vi "Script Project FIFOs.vi"(7 "Number of SPI Buses":i32, 8 "error in (no error)":errorcluster, 9 "Device Channels":i32[](array[numeric]), 10 "LabVIEW Project to Script":path, 11 "Curent Bus Path":path) -> (0 "error out":errorcluster)   [LabVIEW 2014, in "Initialization and IO Node Scripting.lvlib"]
uses:
  Initialization and IO Node Scripting.lvlib
  State Machine/Controls/Values for Naming.ctl
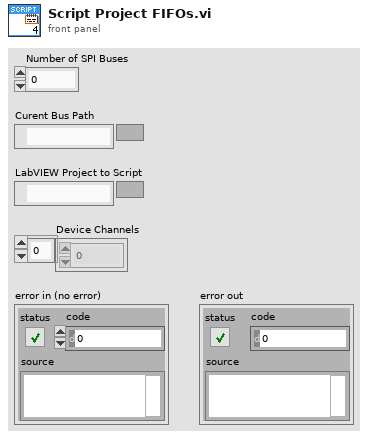
[diagram p1: front panel]
types:
  T1 = typedef "Initialization and IO Node Scripting.lvlib/Values for Naming.ctl" = cluster{"Bus Number":i32, "Device Number":i32, "Channel Number":i32}
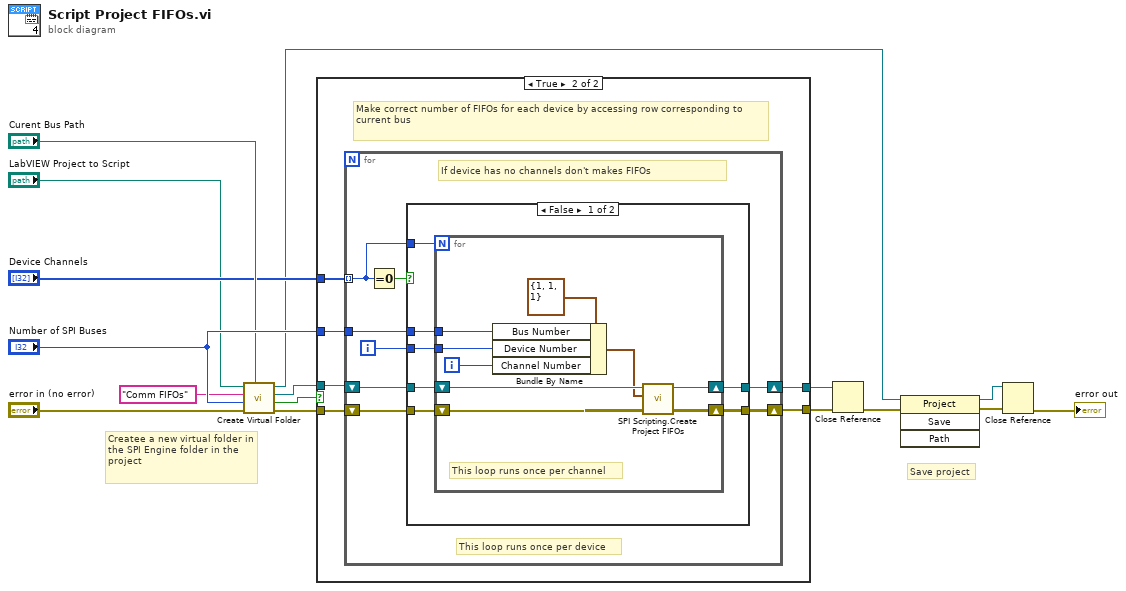
[diagram p0: block diagram]
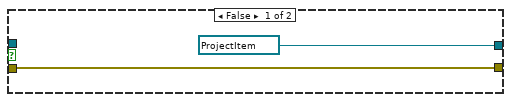
[diagram p2: hidden frame]
diagram:
  # "Save project"
  # "Createe a new virtual folder in the SPI Engine folder in the project"
  n1 = call "Create Virtual Folder.vi"("Curent Bus Path"="Curent Bus Path", "error in"="error in (no error)", "Bus Number"="Number of SPI Buses", "Virtual Folder Name"="Comm FIFOs", "Path to Project"="LabVIEW Project to Script") -> ("error out"=w10:errorcluster, "FPGA Target Found"=w12:bool, "New Virtual Folder"=w13:refnum<vi>, "Project:Open"=w9:refnum<vi>)  [unwired: 3 in]
  n2 = case shown="True" w12 {
    tunnel: [w18 w24] -> w8
    tunnel: w10 -> [w18 w23]
    tunnel: [refnum<vi> refnum ("Comm FIFOs Virtual Folder") w22] -> w11
    tunnel: w13 -> [_ w21]
    tunnel: "Device Channels" -> [_ w19]
    tunnel: "Number of SPI Buses" -> [_ w20]
    frame False {
    }
    frame True {
      # "Make correct number of FIFOs for each device by accessing row corresponding to current bus"
      n3 = for {
        shift-right: [w32] -> w24
        shift-left: w23 -> [w31]
        tunnel: w19 -> [w26] mode=indexing
        shift-right: [w30] -> w22
        shift-left: w21 -> [w29]
        tunnel: w20 -> [w25]
        i -> [w27]
        # "This loop runs once per device"
        # "If device has no channels don't makes FIFOs"
        n4 = Equal To 0?(x=w26) -> (x = 0?=w28:bool)
        n5 = case shown="False" w28 {
          tunnel: [w39 w50] -> w32
          tunnel: w31 -> [w38 w50]
          tunnel: [w37 w49] -> w30
          tunnel: w29 -> [w36 w49]
          tunnel: w27 -> [w35 _]
          tunnel: w26 -> [w34 _]
          tunnel: w25 -> [w33 _]
          frame False {
            n6 = for {
              N: w34 -> [_]
              shift-right: [w48] -> w39
              shift-left: w38 -> [w47]
              shift-right: [w46] -> w37
              shift-left: w36 -> [w45]
              tunnel: w35 -> [w42]
              tunnel: w33 -> [w41]
              i -> [w43]
              # "This loop runs once per channel"
              n7 = Bundle By Name(cluster=T1 {"Bus Number"=1, "Device Number"=1, "Channel Number"=1} ("Values for Naming"), "Bus Number"=w41, "Device Number"=w42, "Channel Number"=w43) -> (w40:T1)
              n8 = call "SPI Scripting.Create Project FIFOs.vi"("error in"=w47, "Values for Naming"=w40, "New Virtual Folder"=w45) -> ("error out"=w48:errorcluster, "Comm FIFOs Virtual Folder"=w46:refnum<vi>)  [unwired: 7 in]
            }
          }
          frame True {
          }
        }
      }
    }
  }
  n9 = Close Reference(reference=w11, error in (no error)=w8) -> (error out=w4:errorcluster)
  n10 = invoke class="Project" method="Save"(reference=w9, error in=w4) -> (reference out=w6:refnum<vi>, error out=w5:errorcluster)  [unwired: 2 in, 2 out]
  n11 = Close Reference(reference=w6, error in (no error)=w5) -> (error out=→"error out":errorcluster)
